vi "gcf_2.vi"(9 "B":i32, 11 "A":i32) -> (3 "GCF":i32)   [LabVIEW 2009]
doc: "Uses the Euclidean algorithm to compute the Greatest Common Factor (Greatest Common Divisor) of two numbers."
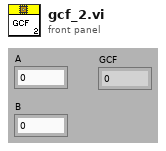
[diagram p1: front panel]
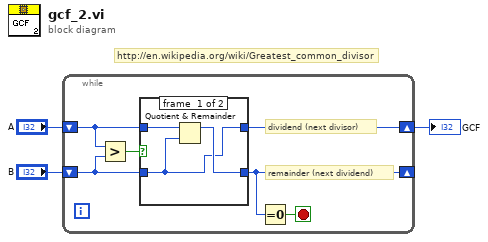
[diagram p0: block diagram]
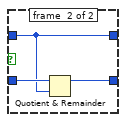
[diagram p2: hidden frame]
diagram:
  # "http://en.wikipedia.org/wiki/Greatest_common_divisor"
  n1 = while {
    shift-right: [w6] -> w1
    shift-left: "A" -> [w8]
    shift-right: [w5] -> _
    shift-left: "B" -> [w7]
    stop <- w4 stop-if-true
    # "dividend (next divisor)"
    # "remainder (next dividend)"
    n2 = Greater?(x=w8, y=w7) -> (0:w9:bool)
    n3 = case shown="False" w9 {
      tunnel: w8 -> [w12 w13]
      tunnel: w7 -> [w10 w14]
      tunnel: [w11 w15] -> w5
      tunnel: [w10 w13] -> w6
      frame #0 {
        n4 = Quotient & Remainder(x=w12, y=w10) -> (x-y*floor(x/y)=w11:i32)  [unwired: 1 out]
      }
      frame #1 {
        n5 = Quotient & Remainder(x=w14, y=w13) -> (x-y*floor(x/y)=w15:i32)  [unwired: 1 out]
      }
    }
    n6 = Equal To 0?(x=w5) -> (x = 0?=w4:bool)
  }
  "GCF" <- w1
